vi "HFRR ADV v11.vi"() -> ()   [LabVIEW 2025] (continued)
              n2114 = String Subset(string=w2524, offset (0)=15, length (rest)=9 ("length (rest)")) -> (substring=w2553:string)
              n2115 = String Subset(string=w2524, offset (0)=0, length (rest)=14 ("length (rest)")) -> (substring=w2550:string)
              n2116 = String Subset(string=w2524, offset (0)=45, length (rest)=9 ("length (rest)")) -> (substring=w2537:string)
              n2117 = String Subset(string=w2524, offset (0)=65, length (rest)=9 ("length (rest)")) -> (substring=w2543:string)
              n2118 = Fract/Exp String To Number(string=w2526) -> (number=w2523:dbl)  [unwired: 3 in, 1 out]
              n2119 = Fract/Exp String To Number(string=w2547) -> (number=w2545:dbl)  [unwired: 3 in, 1 out]
              n2120 = Fract/Exp String To Number(string=w2532) -> (number=w2530:dbl)  [unwired: 3 in, 1 out]
              n2121 = Fract/Exp String To Number(string=w2528) -> (number=w2527:dbl)  [unwired: 3 in, 1 out]
              n2122 = Fract/Exp String To Number(string=w2553) -> (number=w2544:dbl)  [unwired: 3 in, 1 out]
              n2123 = Fract/Exp String To Number(string=w2550) -> (number=w2546:dbl)  [unwired: 3 in, 1 out]
              n2124 = Fract/Exp String To Number(string=w2537) -> (number=w2534:dbl)  [unwired: 3 in, 1 out]
              n2125 = Fract/Exp String To Number(string=w2543) -> (number=w2540:dbl)  [unwired: 3 in, 1 out]
              n2126 = Add(x=w2540, y=0.0) -> (x+y=w2538:dbl)
            }
            n2127 = String To Path(string=w2383) -> (path=w2481:path)
            n2128 = String To Path(string=w2381) -> (path=w2475:path)
            n2129 = local read "Numeric 11"() -> (w2465:i32)
            n2130 = local read "Numeric 13"() -> (w2467:i32)
            n2131 = Open/Create/Replace File "Open File"(file path (use dialog)=w2481) -> (refnum out=w2479:refnum<file>, error out=w2478:errorcluster)  [unwired: 5 in, 1 out]
            n2132 = Open/Create/Replace File "Open File"(file path (use dialog)=w2475) -> (refnum out=w2474:refnum<file>, error out=w2473:errorcluster)  [unwired: 5 in, 1 out]
            n2133 = for {
              N: w2465 -> [_]
              tunnel: w2479 -> [w2594]
              tunnel: w2478 -> [w2593]
              tunnel: [w2583] -> w2445 mode=indexing
              tunnel: [w2581] -> w2443 mode=indexing
              tunnel: [w2582] -> w2438 mode=indexing
              tunnel: w2464 -> [_]
              tunnel: [w2575] -> w2440 mode=indexing
              tunnel: [w2571] -> w2416 mode=indexing
              tunnel: [w2567] -> w2391 mode=indexing
              tunnel: [w2563] -> w2372 mode=indexing
              tunnel: [w2558] -> w2330 mode=indexing
              (unwired) TRUE ("line mode (F)")
              n2134 = Read from Text File "Read File"(file (use dialog)=w2594, error in=w2593) -> (text=w2559:string)  [unwired: 2 in, 3 out]
              n2135 = local write "String 7"(w2559) -> ()
              n2136 = String Subset(string=w2559, offset (0)=85, length (rest)=9 ("length (rest)")) -> (substring=w2562:string)
              n2137 = String Subset(string=w2559, offset (0)=35, length (rest)=9 ("length (rest)")) -> (substring=w2584:string)
              n2138 = String Subset(string=w2559, offset (0)=55, length (rest)=9 ("length (rest)")) -> (substring=w2570:string)
              n2139 = String Subset(string=w2559, offset (0)=25, length (rest)=9 ("length (rest)")) -> (substring=w2564:string)
              n2140 = String Subset(string=w2559, offset (0)=45, length (rest)=9 ("length (rest)")) -> (substring=w2572:string)
              n2141 = String Subset(string=w2559, offset (0)=0, length (rest)=14 ("length (rest)")) -> (substring=w2587:string)
              n2142 = String Subset(string=w2559, offset (0)=15, length (rest)=9 ("length (rest)")) -> (substring=w2590:string)
              n2143 = String Subset(string=w2559, offset (0)=65, length (rest)=9 ("length (rest)")) -> (substring=w2576:string)
              n2144 = Fract/Exp String To Number(string=w2562) -> (number=w2558:dbl)  [unwired: 3 in, 1 out]
              n2145 = Fract/Exp String To Number(string=w2584) -> (number=w2582:dbl)  [unwired: 3 in, 1 out]
              n2146 = Fract/Exp String To Number(string=w2570) -> (number=w2567:dbl)  [unwired: 3 in, 1 out]
              n2147 = Fract/Exp String To Number(string=w2564) -> (number=w2563:dbl)  [unwired: 3 in, 1 out]
              n2148 = Fract/Exp String To Number(string=w2572) -> (number=w2571:dbl)  [unwired: 3 in, 1 out]
              n2149 = Fract/Exp String To Number(string=w2587) -> (number=w2583:dbl)  [unwired: 3 in, 1 out]
              n2150 = Fract/Exp String To Number(string=w2590) -> (number=w2581:dbl)  [unwired: 3 in, 1 out]
              n2151 = Fract/Exp String To Number(string=w2576) -> (number=w2579:dbl)  [unwired: 3 in, 1 out]
              n2152 = Add(x=w2579, y=0.0) -> (x+y=w2575:dbl)
            }
            n2153 = for {
              N: w2467 -> [_]
              tunnel: w2474 -> [w2522]
              tunnel: w2473 -> [w2521]
              tunnel: [w2511] -> w2427 mode=indexing
              tunnel: [w2510] -> w2420 mode=indexing
              tunnel: w2464 -> [_]
              tunnel: [w2499] -> w2425 mode=indexing
              tunnel: [w2504] -> w2422 mode=indexing
              tunnel: [w2500] -> w2412 mode=indexing
              tunnel: [w2495] -> w2387 mode=indexing
              tunnel: [w2491] -> w2368 mode=indexing
              tunnel: [w2486] -> w2328 mode=indexing
              (unwired) 1.0 ("x")
              (unwired) TRUE ("line mode (F)")
              n2154 = Read from Text File "Read File"(file (use dialog)=w2522, error in=w2521) -> (text=w2487:string)  [unwired: 2 in, 3 out]
              n2155 = local write "String 12"(w2487) -> ()
              n2156 = String Subset(string=w2487, offset (0)=85, length (rest)=9 ("length (rest)")) -> (substring=w2489:string)
              n2157 = String Subset(string=w2487, offset (0)=35, length (rest)=9 ("length (rest)")) -> (substring=w2512:string)
              n2158 = String Subset(string=w2487, offset (0)=55, length (rest)=9 ("length (rest)")) -> (substring=w2497:string)
              n2159 = String Subset(string=w2487, offset (0)=25, length (rest)=9 ("length (rest)")) -> (substring=w2493:string)
              n2160 = String Subset(string=w2487, offset (0)=45, length (rest)=9 ("length (rest)")) -> (substring=w2502:string)
              n2161 = String Subset(string=w2487, offset (0)=15, length (rest)=9 ("length (rest)")) -> (substring=w2518:string)
              n2162 = String Subset(string=w2487, offset (0)=0, length (rest)=14 ("length (rest)")) -> (substring=w2515:string)
              n2163 = String Subset(string=w2487, offset (0)=65, length (rest)=9 ("length (rest)")) -> (substring=w2505:string)
              n2164 = Fract/Exp String To Number(string=w2489) -> (number=w2486:dbl)  [unwired: 3 in, 1 out]
              n2165 = Fract/Exp String To Number(string=w2512) -> (number=w2510:dbl)  [unwired: 3 in, 1 out]
              n2166 = Fract/Exp String To Number(string=w2497) -> (number=w2495:dbl)  [unwired: 3 in, 1 out]
              n2167 = Fract/Exp String To Number(string=w2493) -> (number=w2491:dbl)  [unwired: 3 in, 1 out]
              n2168 = Fract/Exp String To Number(string=w2502) -> (number=w2500:dbl)  [unwired: 3 in, 1 out]
              n2169 = Fract/Exp String To Number(string=w2518) -> (number=w2499:dbl)  [unwired: 3 in, 1 out]
              n2170 = Fract/Exp String To Number(string=w2515) -> (number=w2511:dbl)  [unwired: 3 in, 1 out]
              n2171 = Fract/Exp String To Number(string=w2505) -> (number=w2508:dbl)  [unwired: 3 in, 1 out]
              n2172 = Add(x=w2508, y=0.0) -> (x+y=w2504:dbl)
            }
            n2173 = Delete From Array(array=w2370, index=0) -> (array with subset deleted=w2343:dbl[])  [unwired: 1 in, 1 out]
            n2174 = Delete From Array(array=w2433, index=0) -> (array with subset deleted=w2406:dbl[])  [unwired: 1 in, 1 out]
            n2175 = Delete From Array(array=w2413, index=0) -> (array with subset deleted=w2401:dbl[])  [unwired: 1 in, 1 out]
            n2176 = Delete From Array(array=w2431, index=0) -> (array with subset deleted=w2432:dbl[])  [unwired: 1 in, 1 out]
            n2177 = call-poly <vilib>:"Mean.vi"("X"=w2343) -> ("mean"=→"КОФ2 4":dbl)  [unwired: 1 out]
            n2178 = call-poly <vilib>:"Mean.vi"("X"=w2406) -> ("mean"=→"КОФ3":dbl)  [unwired: 1 out]
            n2179 = call-poly <vilib>:"Mean.vi"("X"=w2401) -> ("mean"=→"CP3":dbl)  [unwired: 1 out]
            n2180 = Delete From Array(array=w2395, index=0) -> (array with subset deleted=w2322:dbl[])  [unwired: 1 in, 1 out]
            n2181 = Delete From Array(array=w2334, index=0) -> (array with subset deleted=w2321:dbl[])  [unwired: 1 in, 1 out]
            n2182 = Delete From Array(array=w2374, index=0) -> (array with subset deleted=w2345:dbl[])  [unwired: 1 in, 1 out]
            n2183 = Delete From Array(array=w2452, index=0) -> (array with subset deleted=w2407:dbl[])  [unwired: 1 in, 1 out]
            n2184 = Delete From Array(array=w2418, index=0) -> (array with subset deleted=w2403:dbl[])  [unwired: 1 in, 1 out]
            "array w/ subset deleted" <- w2403
            n2185 = Delete From Array(array=w2449, index=0) -> (array with subset deleted=w2450:dbl[])  [unwired: 1 in, 1 out]
            n2186 = call-poly <vilib>:"Mean.vi"("X"=w2345) -> ("mean"=→"КОФ2 2":dbl)  [unwired: 1 out]
            n2187 = call-poly <vilib>:"Mean.vi"("X"=w2407) -> ("mean"=→"КОФ1":dbl)  [unwired: 1 out]
            n2188 = Bundle "Bundle"(w2322, w2321) -> (w2327:cluster{dbl[], dbl[]})  [unwired: 1 in]
            n2189 = Bundle "Bundle"(w2322, w2450) -> (w2314:cluster{dbl[], dbl[]})  [unwired: 1 in]
            n2190 = Delete From Array(array=w2329, index=0) -> (array with subset deleted=w2317:dbl[])  [unwired: 1 in, 1 out]
            n2191 = Delete From Array(array=w2330, index=0) -> (array with subset deleted=w2319:dbl[])  [unwired: 1 in, 1 out]
            n2192 = Delete From Array(array=w2440, index=0) -> (array with subset deleted=w2441:dbl[])  [unwired: 1 in, 1 out]
            n2193 = Delete From Array(array=w2328, index=0) -> (array with subset deleted=w2315:dbl[])  [unwired: 1 in, 1 out]
            n2194 = Delete From Array(array=w2422, index=0) -> (array with subset deleted=w2423:dbl[])  [unwired: 1 in, 1 out]
            n2195 = Delete From Array(array=w2447, index=0) -> (array with subset deleted=w2353:dbl[])  [unwired: 1 in, 1 out]
            n2196 = Delete From Array(array=w2393, index=0) -> (array with subset deleted=w2349:dbl[])  [unwired: 1 in, 1 out]
            n2197 = Delete From Array(array=w2429, index=0) -> (array with subset deleted=w2351:dbl[])  [unwired: 1 in, 1 out]
            n2198 = Delete From Array(array=w2389, index=0) -> (array with subset deleted=w2347:dbl[])  [unwired: 1 in, 1 out]
            n2199 = Delete From Array(array=w2438, index=0) -> (array with subset deleted=w2352:dbl[])  [unwired: 1 in, 1 out]
            n2200 = Delete From Array(array=w2391, index=0) -> (array with subset deleted=w2348:dbl[])  [unwired: 1 in, 1 out]
            n2201 = Delete From Array(array=w2372, index=0) -> (array with subset deleted=w2344:dbl[])  [unwired: 1 in, 1 out]
            n2202 = Delete From Array(array=w2416, index=0) -> (array with subset deleted=w2402:dbl[])  [unwired: 1 in, 1 out]
            n2203 = Delete From Array(array=w2443, index=0) -> (array with subset deleted=w2404:dbl[])  [unwired: 1 in, 1 out]
            n2204 = Delete From Array(array=w2420, index=0) -> (array with subset deleted=w2350:dbl[])  [unwired: 1 in, 1 out]
            n2205 = Delete From Array(array=w2387, index=0) -> (array with subset deleted=w2346:dbl[])  [unwired: 1 in, 1 out]
            n2206 = Delete From Array(array=w2368, index=0) -> (array with subset deleted=w2342:dbl[])  [unwired: 1 in, 1 out]
            n2207 = Delete From Array(array=w2412, index=0) -> (array with subset deleted=w2400:dbl[])  [unwired: 1 in, 1 out]
            n2208 = Delete From Array(array=w2425, index=0) -> (array with subset deleted=w2405:dbl[])  [unwired: 1 in, 1 out]
            n2209 = Delete From Array(array=w2435, index=0) -> (array with subset deleted=w2318:dbl[])  [unwired: 1 in, 1 out]
            n2210 = Delete From Array(array=w2445, index=0) -> (array with subset deleted=w2320:dbl[])  [unwired: 1 in, 1 out]
            n2211 = Delete From Array(array=w2427, index=0) -> (array with subset deleted=w2316:dbl[])  [unwired: 1 in, 1 out]
            n2212 = Bundle "Bundle"(w2322, w2353) -> (w2340:cluster{dbl[], dbl[]})  [unwired: 1 in]
            n2213 = Bundle "Bundle"(w2322, w2407) -> (w2341:cluster{dbl[], dbl[]})  [unwired: 1 in]
            n2214 = Bundle "Bundle"(w2353, w2349) -> (w2355:cluster{dbl[], dbl[]})  [unwired: 1 in]
            n2215 = Bundle "Bundle"(w2318, w2317) -> (w2325:cluster{dbl[], dbl[]})  [unwired: 1 in]
            n2216 = Bundle "Bundle"(w2351, w2347) -> (w2357:cluster{dbl[], dbl[]})  [unwired: 1 in]
            n2217 = Bundle "Bundle"(w2318, w2351) -> (w2461:cluster{dbl[], dbl[]})  [unwired: 1 in]
            n2218 = Bundle "Bundle"(w2318, w2347) -> (w2385:cluster{dbl[], dbl[]})  [unwired: 1 in]
            n2219 = Bundle "Bundle"(w2318, w2406) -> (w2471:cluster{dbl[], dbl[]})  [unwired: 1 in]
            n2220 = Bundle "Bundle"(w2318, w2401) -> (w2409:cluster{dbl[], dbl[]})  [unwired: 1 in]
            n2221 = Bundle "Bundle"(w2318, w2432) -> (w2456:cluster{dbl[], dbl[]})  [unwired: 1 in]
            n2222 = Bundle "Bundle"(w2352, w2348) -> (w2356:cluster{dbl[], dbl[]})  [unwired: 1 in]
            n2223 = Bundle "Bundle"(w2320, w2319) -> (w2326:cluster{dbl[], dbl[]})  [unwired: 1 in]
            n2224 = Bundle "Bundle"(w2320, w2352) -> (w2463:cluster{dbl[], dbl[]})  [unwired: 1 in]
            n2225 = Bundle "Bundle"(w2320, w2348) -> (w2386:cluster{dbl[], dbl[]})  [unwired: 1 in]
            n2226 = Bundle "Bundle"(w2320, w2402) -> (w2410:cluster{dbl[], dbl[]})  [unwired: 1 in]
            n2227 = Bundle "Bundle"(w2320, w2404) -> (w2472:cluster{dbl[], dbl[]})  [unwired: 1 in]
            n2228 = Bundle "Bundle"(w2320, w2441) -> (w2454:cluster{dbl[], dbl[]})  [unwired: 1 in]
            n2229 = Bundle "Bundle"(w2350, w2346) -> (w2358:cluster{dbl[], dbl[]})  [unwired: 1 in]
            n2230 = Bundle "Bundle"(w2316, w2315) -> (w2324:cluster{dbl[], dbl[]})  [unwired: 1 in]
            n2231 = Bundle "Bundle"(w2316, w2350) -> (w2462:cluster{dbl[], dbl[]})  [unwired: 1 in]
            n2232 = Bundle "Bundle"(w2316, w2346) -> (w2384:cluster{dbl[], dbl[]})  [unwired: 1 in]
            n2233 = Bundle "Bundle"(w2316, w2400) -> (w2408:cluster{dbl[], dbl[]})  [unwired: 1 in]
            n2234 = Bundle "Bundle"(w2316, w2405) -> (w2470:cluster{dbl[], dbl[]})  [unwired: 1 in]
            n2235 = Bundle "Bundle"(w2316, w2423) -> (w2455:cluster{dbl[], dbl[]})  [unwired: 1 in]
            n2236 = call-poly <vilib>:"Mean.vi"("X"=w2403) -> ("mean"=→"CP1":dbl)  [unwired: 1 out]
            n2237 = call-poly <vilib>:"Mean.vi"("X"=w2344) -> ("mean"=→"КОФ2 3":dbl)  [unwired: 1 out]
            n2238 = call-poly <vilib>:"Mean.vi"("X"=w2402) -> ("mean"=→"CP2":dbl)  [unwired: 1 out]
            n2239 = call-poly <vilib>:"Mean.vi"("X"=w2404) -> ("mean"=→"КОФ2":dbl)  [unwired: 1 out]
            n2240 = call-poly <vilib>:"Mean.vi"("X"=w2342) -> ("mean"=→"КОФ2 5":dbl)  [unwired: 1 out]
            n2241 = call-poly <vilib>:"Mean.vi"("X"=w2400) -> ("mean"=→"CP4":dbl)  [unwired: 1 out]
            n2242 = call-poly <vilib>:"Mean.vi"("X"=w2405) -> ("mean"=→"КОФ4":dbl)  [unwired: 1 out]
            n2243 = Bundle "Bundle"(w2322, w2349) -> (w2313:cluster{dbl[], dbl[]})  [unwired: 1 in]
            n2244 = Bundle "Bundle"(w2322, w2403) -> (w2336:cluster{dbl[], dbl[]})  [unwired: 1 in]
            n2245 = Build Array "Build Array"(w2313, w2336) -> (w2339:cluster{dbl[], dbl[]}[])
            "XY Graph 17" <- w2339
            n2246 = Build Array "Build Array"(w2327, w2326, w2325, w2324) -> (→"Frequency ( Hz )":cluster{dbl[], dbl[]}[])
            n2247 = Build Array "Build Array"(w2355, w2356, w2357, w2358) -> (→"Air Temp ( °C ) vs Humidity ( % RH )":cluster{dbl[], dbl[]}[])
            n2248 = Build Array "Build Array"(w2340, w2463, w2461, w2462) -> (→"Air Temperature  ( °C )":cluster{dbl[], dbl[]}[])
            n2249 = Build Array "Build Array"(w2313, w2386, w2385, w2384) -> (→"Humidity ( %RH )":cluster{dbl[], dbl[]}[])
            n2250 = Build Array "Build Array"(w2341, w2472, w2471, w2470) -> (→"Coefficient Of Friction":cluster{dbl[], dbl[]}[])
            n2251 = Build Array "Build Array"(w2336, w2410, w2409, w2408) -> (→"Sample Temperature ( °C )":cluster{dbl[], dbl[]}[])
            n2252 = Build Array "Build Array"(w2314, w2454, w2456, w2455) -> (→"XY Graph 13":cluster{dbl[], dbl[]}[])
            n2253 = Bundle "Bundle"(w2322, w2345) -> (w2367:cluster{dbl[], dbl[]})  [unwired: 1 in]
            n2254 = Bundle "Bundle"(w2318, w2343) -> (w2365:cluster{dbl[], dbl[]})  [unwired: 1 in]
            n2255 = Bundle "Bundle"(w2320, w2344) -> (w2366:cluster{dbl[], dbl[]})  [unwired: 1 in]
            n2256 = Bundle "Bundle"(w2316, w2342) -> (w2364:cluster{dbl[], dbl[]})  [unwired: 1 in]
            n2257 = Build Array "Build Array"(w2367, w2366, w2365, w2364) -> (→"Stroke ( mm )":cluster{dbl[], dbl[]}[])
            n2258 = local write "XY Graph 16"(w2339) -> ()
          }
          frame #2 {
          }
          frame #3 {
            n2259 = local write "Numeric 8"(0 ("Numeric 8")) -> ()
            n2260 = local write "Numeric 11"(0 ("Numeric 11")) -> ()
            n2261 = local write "Numeric 12"(0 ("Numeric 12")) -> ()
            n2262 = local write "Numeric 13"(0 ("Numeric 13")) -> ()
            n2263 = property on="OPEN" class="Bool (strict)"("Visible"=TRUE) -> ()  [unwired: 2 in, 2 out]
            n2264 = local read "String Control 2"() -> (w2639:string)
            n2265 = local read "String Control 4"() -> (w2638:string)
            n2266 = local read "String Control 6"() -> (w2637:string)
            n2267 = local read "String Control 8"() -> (w2636:string)
            n2268 = Match Pattern(string=w2639, regular expression="Samples / cycle :- ") -> (after substring=w2653:string)  [unwired: 1 in, 3 out]
            n2269 = Match Pattern(string=w2639, regular expression="Frequency :- ") -> (after substring=w2672:string)  [unwired: 1 in, 3 out]
            n2270 = Match Pattern(string=w2638, regular expression="Samples / cycle :- ") -> (after substring=w2649:string)  [unwired: 1 in, 3 out]
            n2271 = Match Pattern(string=w2638, regular expression="Frequency :- ") -> (after substring=w2667:string)  [unwired: 1 in, 3 out]
            n2272 = Match Pattern(string=w2637, regular expression="Samples / cycle :- ") -> (after substring=w2645:string)  [unwired: 1 in, 3 out]
            n2273 = Match Pattern(string=w2637, regular expression="Frequency :- ") -> (after substring=w2662:string)  [unwired: 1 in, 3 out]
            n2274 = Match Pattern(string=w2636, regular expression="Samples / cycle :- ") -> (after substring=w2641:string)  [unwired: 1 in, 3 out]
            n2275 = Match Pattern(string=w2636, regular expression="Frequency :- ") -> (after substring=w2657:string)  [unwired: 1 in, 3 out]
            n2276 = String Subset(string=w2653, length (rest)=6 ("length (rest)")) -> (substring=w2655:string)  [unwired: 1 in]
            n2277 = String Subset(string=w2672, length (rest)=9 ("length (rest)")) -> (substring=w2674:string)  [unwired: 1 in]
            n2278 = String Subset(string=w2649, length (rest)=6 ("length (rest)")) -> (substring=w2651:string)  [unwired: 1 in]
            n2279 = String Subset(string=w2667, length (rest)=9 ("length (rest)")) -> (substring=w2669:string)  [unwired: 1 in]
            n2280 = String Subset(string=w2645, length (rest)=6 ("length (rest)")) -> (substring=w2647:string)  [unwired: 1 in]
            n2281 = String Subset(string=w2662, length (rest)=9 ("length (rest)")) -> (substring=w2664:string)  [unwired: 1 in]
            n2282 = String Subset(string=w2641, length (rest)=6 ("length (rest)")) -> (substring=w2643:string)  [unwired: 1 in]
            n2283 = String Subset(string=w2657, length (rest)=9 ("length (rest)")) -> (substring=w2659:string)  [unwired: 1 in]
            n2284 = Fract/Exp String To Number(string=w2655) -> (number=w2635:dbl)  [unwired: 3 in, 1 out]
            n2285 = Fract/Exp String To Number(string=w2674) -> (number=w2675:dbl)  [unwired: 3 in, 1 out]
            n2286 = Fract/Exp String To Number(string=w2651) -> (number=w2634:dbl)  [unwired: 3 in, 1 out]
            n2287 = Fract/Exp String To Number(string=w2669) -> (number=w2670:dbl)  [unwired: 3 in, 1 out]
            n2288 = Fract/Exp String To Number(string=w2647) -> (number=w2633:dbl)  [unwired: 3 in, 1 out]
            n2289 = Fract/Exp String To Number(string=w2664) -> (number=w2665:dbl)  [unwired: 3 in, 1 out]
            n2290 = Fract/Exp String To Number(string=w2643) -> (number=w2632:dbl)  [unwired: 3 in, 1 out]
            n2291 = Fract/Exp String To Number(string=w2659) -> (number=w2660:dbl)  [unwired: 3 in, 1 out]
            n2292 = local write "sample1"(w2635) -> ()
            n2293 = local write "freq1"(w2675) -> ()
            n2294 = local write "sample2"(w2634) -> ()
            n2295 = local write "freq2"(w2670) -> ()
            n2296 = local write "sample3"(w2633) -> ()
            n2297 = local write "freq3"(w2665) -> ()
            n2298 = local write "sample4"(w2632) -> ()
            n2299 = local write "freq 4"(w2660) -> ()
          }
        }
      }
    }
    n2300 = case shown="True" w2122 {
      selector: w2122 -> [_ w2251]
      frame False {
      }
      frame True {
        n2301 = Not(x=w2251) -> (.not. x?=w2247:bool)
        n2302 = local write "service 3"(w2247) -> ()
        n2303 = local write "OPEN 6"(w2247) -> ()
        n2304 = call <vilib>:"System Exec.vi"("wait until completion? (T)"=TRUE, "command line"="C:\\LAB-IQ\\Scar View.exe") -> ("error out"=→"error out 5":errorcluster)  [unwired: 6 in, 3 out]
      }
    }
    n2305 = case shown="\"Acquire\", Default" w2134 {
      frame "Acquire", Default {
        w3174 = 0.2 ("y")
        w3179 = 1.0 ("y")
        w3180 = 0.8 ("y")
        # "Elapsed time\ncof\nstroke\nAir temp\nTemp\nHumidity"
        n2306 = disable-structure shown="Disabled" {
          frame Disabled {
            n2307 = local read "Flag"() -> (w3197:dbl)
            n2308 = local read "RUN"() -> (w3194:bool)
            n2309 = Not(x=w3194) -> (.not. x?=w3193:bool)
            n2310 = Equal?(x=w3197, y=10.0) -> (x = y?=w3195:bool)
            n2311 = And(x=w3195, y=w3193) -> (x .and. y?=w3192:bool)
            n2312 = case shown="True" w3192 {
              frame False {
              }
              frame True {
                w3198 = FALSE ("Heater Button")
                n2313 = local write "Humidity"(w3198) -> ()
                n2314 = local write "Heater Button"(w3198) -> ()
              }
            }
          }
          frame Enabled {
          }
        }
        n2315 = disable-structure shown="Disabled" {
          frame Disabled {
            n2316 = case shown="True" {
              selector: _ -> [_ _]
              frame False {
              }
              frame True {
                w3289 = TRUE ("Heater")
                n2317 = local write "Humidity"(w3289) -> ()
                n2318 = local write "Heater Button"(w3289) -> ()
                n2319 = local read "TEST STANDARD"() -> (w3292:T3)
                n2320 = local read "TEST STANDARD"() -> (w3287:T3)
                n2321 = Equal?(x=w3292, y=enum16{"ASTM D6079", "ISO 12156", "Custom"}."ISO 12156" ("Test Standard")) -> (x = y?=w3290:bool)
                n2322 = Equal?(x=w3287, y=enum16{"ASTM D6079", "ISO 12156", "Custom"}."ASTM D6079" ("Test Standard")) -> (x = y?=w3286:bool)
                n2323 = case shown="True" w3290 {
                  frame False {
                  }
                  frame True {
                    n2324 = local write "Heater"(TRUE ("Heater")) -> ()
                    n2325 = local write "airtempflg"(FALSE ("airtempflg")) -> ()
                  }
                }
                n2326 = case shown="True" w3286 {
                  frame False {
                  }
                  frame True {
                    n2327 = local write "Heater"(FALSE ("Heater")) -> ()
                    n2328 = local write "airtempflg"(TRUE ("airtempflg")) -> ()
                  }
                }
              }
            }
          }
          frame Enabled {
          }
        }
        n2329 = stacked-sequence {
          frame #0 {
            n2330 = case shown="True" "RST FF" {
              frame False {
              }
              frame True {
                w3355 = 0.0 ("X Scale.Range:Maximum")
                n2331 = property on="Frictional Force ( N )" class="WFChart (strict)"("XScale.Maximum"=600.0 ("X Scale.Range:Maximum"), "XScale.Minimum"=w3355, "YScale.Maximum"=10.0 ("Y Scale.Range:Maximum"), "YScale.Minimum"=w3355) -> ()  [unwired: 2 in, 2 out]
              }
            }
          }
          frame #1 {
            n2332 = case shown="True" "RST TEMP" {
              frame False {
              }
              frame True {
                n2333 = property on="Temperature ( Deg C )" class="WFChart (strict)"("XScale.Minimum"=0.0 ("X Scale.Range:Minimum"), "XScale.Maximum"=600.0 ("X Scale.Range:Maximum"), "YScale.Minimum"=0.0 ("Y Scale.Range:Minimum"), "YScale.Maximum"=100.0 ("Y Scale.Range:Maximum")) -> ()  [unwired: 2 in, 2 out]
              }
            }
          }
          frame #2 {
            n2334 = case shown="True" "RSTCOF" {
              frame False {
              }
              frame True {
                n2335 = property on="Coefficient of Friction" class="WFChart (strict)"("XScale.Minimum"=0.0 ("X Scale.Range:Minimum"), "XScale.Maximum"=600.0 ("X Scale.Range:Maximum"), "YScale.Maximum"=1.0 ("X Scale.Range:Minimum"), "YScale.Minimum"=0.0 ("X Scale.Range:Minimum")) -> ()  [unwired: 2 in, 2 out]
              }
            }
          }
          frame #3 {
            n2336 = case shown="True" "RSTCOF 2" {
              frame False {
              }
              frame True {
                (unwired) 100.0 ("Y Scale.Range:Maximum")
                (unwired) 0.0 ("Y Scale.Range:Minimum")
                (unwired) 600.0 ("X Scale.Range:Maximum")
                (unwired) 0.0 ("X Scale.Range:Minimum")
              }
            }
          }
          frame #4 {
            n2337 = case shown="True" "RSTCOF 3" {
              frame False {
              }
              frame True {
                n2338 = property on="Electrical Contact Resistance ( % )" class="WFChart (strict)"("XScale.Minimum"=0.0 ("X Scale.Range:Minimum"), "XScale.Maximum"=600.0 ("X Scale.Range:Maximum"), "YScale.Minimum"=0.0 ("Y Scale.Range:Minimum"), "YScale.Maximum"=100.0 ("Y Scale.Range:Maximum")) -> ()  [unwired: 2 in, 2 out]
              }
            }
          }
        }
        n2339 = disable-structure shown="Disabled" {
          frame Disabled {
            n2340 = case shown="True" {
              selector: _ -> [_ _]
              frame False {
              }
              frame True {
                n2341 = local read "zflag 2"() -> (w3256:dbl)
                n2342 = local read "yflag"() -> (w3258:dbl)
                n2343 = Equal?(x=w3258, y=2.0 ("tflag")) -> (x = y?=w3260:bool)
                n2344 = Equal?(x=w3256, y=3.0 ("tflag")) -> (x = y?=w3259:bool)
                n2345 = And(x=w3260, y=w3259) -> (x .and. y?=w3254:bool)
                n2346 = case shown="True" w3254 {
                  frame False {
                  }
                  frame True {
                    w3285 = 0.0 ("zflag")
                    n2347 = local write "zflag"(w3285) -> ()
                    n2348 = local write "zflag 2"(w3285) -> ()
                    n2349 = Delete(path (use dialog)=path "C:/LAB-IQ-NXT/WO 2449 TT.sig" ("file path (dialog if empty)")) -> (deleted path=w3284:path)  [unwired: 4 in, 2 out]
                    n2350 = Delete(path (use dialog)=path "C:/LAB-IQ-NXT/WO 2449 TRH.sig" ("file path (dialog if empty)")) -> (deleted path=w3279:path)  [unwired: 4 in, 2 out]
                    n2351 = local read "SEN.RUN HRS"() -> (w3271:dbl)
                    n2352 = local read "SENSOR TIME"() -> (w3269:dbl)
                    n2353 = call <vilib>:"compatOverwrite.vi"("overwrite (F)"=TRUE) -> ("overwrite?"=w3261:T26)
                    n2354 = call <vilib>:"compatOverwrite.vi"("overwrite (F)"=TRUE) -> ("overwrite?"=w3265:T26)
                    n2355 = local read "Total No. of Tests"() -> (w3272:dbl)
                    n2356 = Add(x=w3269, y=w3271) -> (x+y=w3270:dbl)
                    "SEN.RUN HRS" <- w3270
                    n2357 = Open/Create/Replace File(file path (use dialog)=w3284, operation (0:open)=w3261) -> (refnum out=w3262:refnum<file>, error out=w3263:errorcluster)  [unwired: 4 in, 1 out]
                    n2358 = Open/Create/Replace File(file path (use dialog)=w3279, operation (0:open)=w3265) -> (refnum out=w3266:refnum<file>, error out=w3267:errorcluster)  [unwired: 4 in, 1 out]
                    n2359 = Deny Access(4:w3263, 6:T24."deny none" ("deny mode (2)"), 7:w3262) -> (3:w3283:refnum<file>)  [unwired: 1 out]
                    n2360 = Deny Access(4:w3267, 6:T24."deny none" ("deny mode (2)"), 7:w3266) -> (3:w3275:refnum<file>)  [unwired: 1 out]
                    n2361 = Number To Decimal String(number=w3272) -> (decimal integer string=w3280:string)  [unwired: 1 in]
                    n2362 = Number To Decimal String(number=w3270) -> (decimal integer string=w3276:string)  [unwired: 1 in]
                    n2363 = Write to Binary File(file (use dialog)=w3283, data=w3280, 5:FALSE ("prepend array or string size? (T)")) -> ()  [unwired: 3 in, 3 out]
                    n2364 = Write to Binary File(file (use dialog)=w3275, data=w3276, 5:FALSE ("prepend array or string size? (T)")) -> ()  [unwired: 3 in, 3 out]
                  }
                }
              }
            }
          }
          frame Enabled {
          }
        }
        n2365 = local read "RUN"() -> (w3183:bool)
        n2366 = local read "run replace"() -> (w3187:bool)
        n2367 = local read "run replace"() -> (w3186:bool)
        n2368 = case shown="True" w3183 {
          frame False {
            n2369 = local write "run replace"(FALSE ("run replace")) -> ()
          }
          frame True {
            "run replace" <- TRUE ("run replace")
          }
        }
        n2370 = local read "RUN"() -> (w3191:bool)
        n2371 = local read "Set Temp"() -> (w3153:dbl)
        n2372 = local read "SetTemp"() -> (w3155:dbl)
        n2373 = case shown="False" w3191 {
          tunnel: [FALSE ("TEST RUNNING") TRUE ("TEST RUNNING")] -> w3190
          frame False {
            w3374 = 0.0 ("Flag")
            n2374 = local write "Elapsed time"(0.0 ("elapsedtime")) -> ()
            n2375 = local write "Time Remaining"(w3374) -> ()
            n2376 = local write "Flag"(w3374) -> ()
            n2377 = local write "Remaining Time"(w3374) -> ()
          }
          frame True {
            n2378 = local write "Flag"(10.0 ("Flag")) -> ()
          }
        }
        n2379 = case shown="False" w3187 {
          frame False {
            n2380 = local read "zflag"() -> (→"zflag 2":dbl)
            n2381 = local write "yflag"(2.0 ("tflag")) -> ()
            n2382 = local write "FLAG 4"(0.0 ("FLAG")) -> ()
          }
          frame True {
            n2383 = local write "yflag"(1.0 ("tflag")) -> ()
            n2384 = local write "zflag"(3.0 ("zflag")) -> ()
          }
        }
        n2385 = local read "acq 2"() -> (w3185:bool)
        n2386 = local read "AIR TEMP"() -> (w3148:dbl)
        n2387 = local read "Amb temp"() -> (w3152:dbl)
        n2388 = case shown="True" "Save & Continue" {
          frame False {
          }
          frame True {
            "acq 2" <- TRUE ("acq 2")
          }
        }
        n2389 = local read "Set Rh"() -> (w3154:dbl)
        n2390 = Add(x=w3155, y=w3180) -> (x+y=w3181:dbl)
        n2391 = Subtract(x=w3155, y=w3180) -> (x-y=w3182:dbl)
        n2392 = Add(x=w3153, y=w3174) -> (x+y=w3175:dbl)
        n2393 = Subtract(x=w3153, y=w3174) -> (x-y=w3176:dbl)
        n2394 = And(x=w3185, y=w3186) -> (x .and. y?=w3184:bool)
        n2395 = Greater Or Equal?(x=w3148, y=15.0) -> (x >= y?=w3149:bool)
        "powstat" <- w3149
        n2396 = local read "Humidity ( %RH )"() -> (w3151:dbl)
        n2397 = case shown="True" "Save & Continue" {
          frame False {
          }
          frame True {
            n2398 = while {
              tunnel: "0123456789abcdefghijklmnopqrstuvwxyzABCDEFGHIJKLMNOPQRSTUVWXYZ" ("string 2") -> [w3345]
              shift-right: [w3343] -> w3338
              shift-left: "" -> [w3342]
              i -> [w3352]
              stop <- w3351 stop-if-true
              n2399 = Random Number (0-1)() -> (number: 0 to 1=w3346:dbl)
              n2400 = Multiply(x=w3346, y=62.0) -> (x*y=w3348:dbl)
              n2401 = Decrement(x="Length") -> (x-1=w3341:i16)
              n2402 = To Word Integer(number=w3348) -> (16bit integer=w3349:i16)
              n2403 = String Subset(string=w3345, offset (0)=w3349, length (rest)=1 ("length (rest)")) -> (substring=w3344:string)
              n2404 = Greater Or Equal?(x=w3352, y=w3341) -> (x >= y?=w3351:bool)
              n2405 = Concatenate Strings(w3344, w3342) -> (w3343:string)
            }
            n2406 = local write "UUID"(w3338) -> ()
          }
        }
        n2407 = In Range and Coerce(upper limit=w3181, x=w3152, lower limit=w3182) -> (In Range?=w3171:bool)  [unwired: 1 out]
        n2408 = Add(x=w3154, y=w3179) -> (x+y=w3178:dbl)
        n2409 = Subtract(x=w3154, y=w3179) -> (x-y=w3177:dbl)
        n2410 = local read "TEMP"() -> (w3150:dbl)
        n2411 = case shown="True" "Save & Continue" {
          frame False {
          }
          frame True {
            n2412 = local read "Operator ID"() -> (w3694:string)
            n2413 = local read "FILE"() -> (w3700:string)
            n2414 = String Length(string=w3700) -> (length=w3698:i32)
            n2415 = String Length(string=w3694) -> (length=w3695:i32)
            n2416 = Greater?(x=w3698, y=0) -> (0:w3697:bool)
            n2417 = Greater?(x=w3695, y=0) -> (0:w3693:bool)
            n2418 = And(x=w3697, y=w3693) -> (x .and. y?=w3692:bool)
            n2419 = case shown="True" w3692 {
              frame False {
                n2420 = stacked-sequence {
                  frame #0 {
                    n2421 = One Button Dialog(message="Please Enter a File Name and Operator ID to save data !", button name ("OK")="Ok") -> ()  [unwired: 1 out]
                  }
                  frame #1 {
                    n2422 = local write "Save & Continue"(FALSE ("OK Button")) -> ()
                  }
                }
                n2423 = local write "Save & Continue"(FALSE ("OK Button")) -> ()
              }
              frame True {
                n2424 = stacked-sequence {
                  frame #0 {
                    n2425 = local read "FILE"() -> (w3706:string)
                    n2426 = call "file check.vi"("file name in"=w3706) -> ("file name out"=w3705:string)  [unwired: 9 in, 1 out]
                    n2427 = call <vilib>:"Application Directory.vi"() -> ("Application Directory"=w3716:path)
                    n2428 = Build Path(base path=w3716, name or relative path="data") -> (appended path=w3715:path)
                    n2429 = call <vilib>:"Trim Whitespace.vi"("string"=w3705) -> ("trimmed string"=w3713:string)  [unwired: 1 in]
                    n2430 = call <vilib>:"Trim Whitespace.vi"("string"=w3705) -> ("trimmed string"=w3714:string)  [unwired: 1 in]
                    n2431 = List Folder(path=w3715) -> (folder names=w3711:string[])  [unwired: 3 in, 3 out]
                    n2432 = Match Pattern(string=w3713, regular expression="_(") -> (before substring=w3710:string)  [unwired: 1 in, 3 out]
                    n2433 = for {
                      tunnel: w3711 -> [w3725] mode=indexing
                      tunnel: w3710 -> [w3723]
                      shift-right: [w3721] -> w3708
                      shift-left: bool[] [] -> [w3722]
                      n2434 = Match Pattern(string=w3725, regular expression="_(") -> (before substring=w3724:string)  [unwired: 1 in, 3 out]
                      n2435 = Equal?(x=w3724, y=w3723) -> (x = y?=w3720:bool)
                      n2436 = case shown="True" w3720 {
                        tunnel: w3720 -> [_ w3728]
                        tunnel: w3722 -> [w3727 w3730]
                        tunnel: [w3727 w3729] -> w3721
                        frame False {
                        }
                        frame True {
                          n2437 = Insert Into Array(array=w3730, new element=w3728) -> (w3729:bool[])  [unwired: 1 in]
                        }
                      }
                    }
                    n2438 = Equal?(x=w3711, y=w3710) -> (x = y?=w3719:bool[])
                    n2439 = Or Array Elements(Boolean array=w3719) -> (logical OR=w3718:bool)
                    n2440 = Array Size(array=w3708) -> (size(s)=w3707:i32)
                    n2441 = case shown="True" w3718 {
                      tunnel: w3714 -> [_ w3738]
                      tunnel: w3707 -> [_ w3731]
                      frame False {
                      }
                      frame True {
                        n2442 = Number To Decimal String(number=w3731) -> (decimal integer string=w3734:string)  [unwired: 1 in]
                        n2443 = Search/Split String(string=w3738, search string/char (-)="_(" ("regular expression")) -> (substring before match=w3736:string)  [unwired: 1 in, 2 out]
                        n2444 = Concatenate Strings(w3736, "_(" ("regular expression"), w3734, ")" ("regular expression")) -> (w3732:string)
                        n2445 = local write "FILE"(w3732) -> ()
                      }
                    }
                  }
                  frame #1 {
                    w3740 = 0.0
                    w3753 = cluster{"y":dbl, dbl, "y":dbl}[] [] ("History Data")
                    w3754 = FALSE ("Heater Button")
                    (unwired) ")!" ("string")
                    (unwired) ")" ("string")
                    w3752 = dbl[] [] ("History Data")
                    w3758 = "\r"
                    # "C:\\WinDucom\\Data\\"
                    # "C:\\LAB-IQ-NXT\\data"
                    n2446 = local write "Humidity ( %RH )"(w3740) -> ()
                    n2447 = local write "Frequency ( Hz )"(w3740) -> ()
                    n2448 = local write "Stroke 3"(w3740) -> ()
                    n2449 = local write "speedop"(0.0 ("PIDclk 2")) -> ()
                    n2450 = local write "Set Temp 2"(65.0 ("Set Temp 2")) -> ()
                    n2451 = local write "AIR TEMP"(w3740) -> ()
                    n2452 = local write "clk"(0.0 ("clk")) -> ()
                    n2453 = local write "Stroke 4"(w3740) -> ()
                    n2454 = local write "Stroke"(w3740) -> ()
                    n2455 = local write "COF 3"(w3740) -> ()
                    n2456 = local write "COF 2"(w3740) -> ()
                    n2457 = local write "TEMP"(w3740) -> ()
                    n2458 = local write "ecr 3"(w3740) -> ()
                    n2459 = local write "FF 3"(w3740) -> ()
                    n2460 = local write "FF 2"(w3740) -> ()
                    n2461 = property on="Humidity ( %RH )" class="WFChart (strict)"("History Data"=w3752) -> ()  [unwired: 2 in, 2 out]
                    n2462 = property on="Coefficient of Friction" class="WFChart (strict)"("History Data"=w3752) -> ()  [unwired: 2 in, 2 out]
                    n2463 = property on="Coefficient of Friction" class="WFChart (strict)"("History Data"=w3752) -> ()  [unwired: 2 in, 2 out]
                    n2464 = property on="Frictional Force ( N )" class="WFChart (strict)"("History Data"=w3752) -> ()  [unwired: 2 in, 2 out]
                    n2465 = property on="Electrical Contact Resistance ( % )" class="WFChart (strict)"("History Data"=w3752) -> ()  [unwired: 2 in, 2 out]
                    n2466 = property on="Electrical Contact Resistance ( % )" class="WFChart (strict)"("History Data"=w3752) -> ()  [unwired: 2 in, 2 out]
                    n2467 = property on="Temperature ( Deg C )" class="WFChart (strict)"("History Data"=w3752) -> ()  [unwired: 2 in, 2 out]
                    n2468 = property on="Frictional Force ( N )" class="WFChart (strict)"("History Data"=w3752) -> ()  [unwired: 2 in, 2 out]
                    n2469 = property on="Coefficient of Friction" class="WFChart (strict)"("History Data"=w3752) -> ()  [unwired: 2 in, 2 out]
                    n2470 = property on="Frictional Force ( N )" class="WFChart (strict)"("History Data"=w3752) -> ()  [unwired: 2 in, 2 out]
                    n2471 = property on="Electrical Contact Resistance ( % )" class="WFChart (strict)"("History Data"=w3752) -> ()  [unwired: 2 in, 2 out]
                    n2472 = property on="Temperature ( Deg C )" class="WFChart (strict)"("History Data"=w3752) -> ()  [unwired: 2 in, 2 out]
                    n2473 = property on="Humidity ( %RH )" class="WFChart (strict)"("History Data"=w3752) -> ()  [unwired: 2 in, 2 out]
                    n2474 = property on="Stroke ( mm )" class="WFChart (strict)"("History Data"=w3753) -> ()  [unwired: 2 in, 2 out]
                    n2475 = property on="Stroke ( mm )" class="WFChart (strict)"("History Data"=w3753) -> ()  [unwired: 2 in, 2 out]
                    n2476 = local write "Humidity"(w3754) -> ()
                    n2477 = local write "Heater Button"(w3754) -> ()
                    n2478 = local read "FILE"() -> (w3748:string)
                    n2479 = disable-structure shown="Enabled" {
                      disable-tunnel: [w3793 _] -> w3739
                      frame Enabled {
                        n2480 = local read "NORMAL LOAD"() -> (w3793:dbl)
                      }
                      frame Disabled {
                      }
                    }
                    n2481 = call "file check.vi"("file name in"=w3748) -> ("error out"=w3751:errorcluster, "file name out"=w3745:string)  [unwired: 9 in]
                    n2482 = call "FILE PATH CREATION.vi"("error in"=w3751, "FILE NAME :"=w3745) -> ("FILE OUT"=w3744:path)  [unwired: 8 in, 1 out]
                    n2483 = Concatenate Strings(w3745, ".dgf" ("Substring")) -> (w3750:string)
                    n2484 = Concatenate Strings(w3745, ".duf" ("Substring")) -> (w3746:string)
                    n2485 = Multiply(x=w3739, y=1.0) -> (x*y=w3772:dbl)
                    n2486 = Build Path(base path=w3744, name or relative path=w3750) -> (appended path=w3743:path)
                    n2487 = Build Path(base path=w3744, name or relative path=w3746) -> (appended path=w3742:path)
                    n2488 = Number To Fractional String(number=w3772, width (-)=i16 5, precision (6)=i16 2) -> (F-format string=w3780:string)  [unwired: 1 in]
                    n2489 = local read "Fuel Discription :"() -> (w3768:string)
                    n2490 = local read "Batch Ref Num :"() -> (w3756:string)
                    n2491 = Get Date/Time String(date format (0)=enum16{"short", "long", "abbreviated"}."short") -> (date string=w3791:string, time string=w3788:string)  [unwired: 2 in]
                    n2492 = local read "Remarks :"() -> (w3767:string)
                    n2493 = Concatenate Strings("Load :- " ("Substring"), w3780, " grams ," ("Substring")) -> (w3779:string)
                    n2494 = local read "String 41"() -> (w3759:string)
                    n2495 = Concatenate Strings(w3768) -> (w3769:string)
                    n2496 = Concatenate Strings(w3756) -> (w3755:string)
                    n2497 = Concatenate Strings("tested by") -> (w3763:string)
                    n2498 = Concatenate Strings("(" ("Substring"), w3791, ")" ("Substring"), w3788) -> (w3761:string)
                    "concatenated string" <- w3761
                    n2499 = Concatenate Strings(w3767, "," ("string")) -> (w3766:string)
                    n2500 = Concatenate Strings("  TIME;      COF;       STROKE;     AIR TEMP;  TEMP;  HUMIDITY;  ECR; PID-OUT; FREQUENCY" ("Substring"), "\r") -> (w3775:string)
                    n2501 = Concatenate Strings(w3759, w3758, "Fuel Discription :-" ("Substring"), w3769, w3758, w3779, w3758, "Batch Ref Num :-" ("Substring"), w3755, w3758, " Remarks :- " ("Substring"), w3766, w3758, " Date :- " ("Substring"), w3761, w3758, "Tested By :-" ("Substring"), w3763) -> (w3773:string)
                    "REMARKS" <- w3773
                    n2502 = call <vilib>:"Write Characters To File.vi"("append to file? (new file:F)"=FALSE, "character string"=w3775, "file path (dialog if empty)"=w3743) -> ()  [unwired: 2 in, 1 out]
                    n2503 = call <vilib>:"Write Characters To File.vi"("append to file? (new file:F)"=FALSE, "character string"=w3773, "file path (dialog if empty)"=w3742) -> ()  [unwired: 2 in, 1 out]
                  }
                  frame #2 {
                    n2504 = local write "Cycles elapsed"(0 ("Cycles elapsed")) -> ()
                    n2505 = local write "cyclecount"(0 ("cyclecount")) -> ()
                    n2506 = local write "Save & Continue"(FALSE ("OK")) -> ()
                    n2507 = local write "autostrtflg"(TRUE ("autostrtflg")) -> ()
                    n2508 = local write "Save"(FALSE ("Save")) -> ()
                    n2509 = Get Date/Time In Seconds() -> (seconds since 1Jan1904=w3798:timestamp)
                    n2510 = To Double Precision Float(number=w3798) -> (double precision float=w3797:dbl)
                    n2511 = local write "acq timer"(w3797) -> ()
                    n2512 = One Button Dialog(message="Please ensure sample is mounted properly and machine is ready in all aspects for testing !", button name ("OK")="Ok") -> ()  [unwired: 1 out]
                  }
                  frame #3 {
                    n2513 = stacked-sequence {
                      frame #0 {
                        n2514 = local write "Main Dashboard Buttons"(T1."Dashboard" ("Main Dashboard Buttons")) -> ()
                        n2515 = local write "Main Tab"(T2."Acquire" ("Main Tab")) -> ()
                      }
                      frame #1 {
                        n2516 = local write "EVENT LOG"("" ("EVENT LOG")) -> ()
                      }
                      frame #2 {
                        n2517 = Wait (ms)(milliseconds to wait=u32 50) -> ()  [unwired: 1 out]
                      }
                      frame #3 {
                        n2518 = disable-structure shown="Disabled" {
                          frame Disabled {
                            n2519 = local read "EVENT LOG"() -> (w3810:string)
                            n2520 = call "Event Log.vi"("Content"="Test Details", "EVENT LOG"=w3810) -> ("EVENT LOG"=w3809:string)  [unwired: 8 in, 1 out]
                            n2521 = local write "EVENT LOG"(w3809) -> ()
                          }
                          frame Enabled {
                          }
                        }
                      }
                      frame #4 {
                        n2522 = Wait (ms)(milliseconds to wait=u32 50) -> ()  [unwired: 1 out]
                      }
                      frame #5 {
                        n2523 = local read "FILE"() -> (w3812:string)
                        n2524 = Concatenate Strings("File Name :" ("Content"), w3812) -> (w3813:string)
                        n2525 = local read "EVENT LOG"() -> (w3816:string)
                        n2526 = call "Event Log.vi"("Content"=w3813, "EVENT LOG"=w3816) -> ("EVENT LOG"=w3815:string)  [unwired: 8 in, 1 out]
                        n2527 = local write "EVENT LOG"(w3815) -> ()
                      }
                      frame #6 {
                        n2528 = Wait (ms)(milliseconds to wait=u32 50) -> ()  [unwired: 1 out]
                      }
                      frame #7 {
                        n2529 = local read "Batch Ref Num :"() -> (w3818:string)
                        n2530 = Concatenate Strings("Batch Ref No :" ("Content"), w3818) -> (w3819:string)
                        n2531 = local read "EVENT LOG"() -> (w3822:string)
                        n2532 = call "Event Log.vi"("Content"=w3819, "EVENT LOG"=w3822) -> ("EVENT LOG"=w3821:string)  [unwired: 8 in, 1 out]
                        n2533 = local write "EVENT LOG"(w3821) -> ()
                      }
                      frame #8 {
                        n2534 = Wait (ms)(milliseconds to wait=u32 50) -> ()  [unwired: 1 out]
                      }
                      frame #9 {
                        n2535 = local read "tested by"() -> (w3824:string)
                        n2536 = Concatenate Strings("Tested By :" ("Content"), w3824) -> (w3825:string)
                        n2537 = local read "EVENT LOG"() -> (w3828:string)
                        n2538 = call "Event Log.vi"("Content"=w3825, "EVENT LOG"=w3828) -> ("EVENT LOG"=w3827:string)  [unwired: 8 in, 1 out]
                        n2539 = local write "EVENT LOG"(w3827) -> ()
                      }
                      frame #10 {
                        n2540 = Wait (ms)(milliseconds to wait=u32 50) -> ()  [unwired: 1 out]
                      }
                      frame #11 {
                        n2541 = local read "TEST STANDARD"() -> (w3831:T3)
                        n2542 = case shown="\"ASTM D6079\", Default" w3831 {
                          tunnel: ["ASTM D6079" "ISO 12156" "CEC F-096-A-06" "Custom"] -> w3830
                          frame "ASTM D6079", Default {
                          }
                          frame "ISO 12156" {
                          }
                          frame "CEC F-096-A-06" {
                          }
                          frame "Custom" {
                          }
                        }
                        n2543 = Concatenate Strings("Test Standard :" ("Content"), w3830) -> (w3832:string)
                        n2544 = local read "EVENT LOG"() -> (w3835:string)
                        n2545 = call "Event Log.vi"("Content"=w3832, "EVENT LOG"=w3835) -> ("EVENT LOG"=w3834:string)  [unwired: 8 in, 1 out]
                        n2546 = local write "EVENT LOG"(w3834) -> ()
                      }
                      frame #12 {
                        n2547 = Wait (ms)(milliseconds to wait=u32 50) -> ()  [unwired: 1 out]
                      }
                      frame #13 {
                        n2548 = local read "Fuel Discription :"() -> (w3841:string)
                        n2549 = Concatenate Strings("Fuel Description :" ("Content"), w3841) -> (w3842:string)
                        n2550 = local read "EVENT LOG"() -> (w3845:string)
                        n2551 = call "Event Log.vi"("Content"=w3842, "EVENT LOG"=w3845) -> ("EVENT LOG"=w3844:string)  [unwired: 8 in, 1 out]
                        n2552 = local write "EVENT LOG"(w3844) -> ()
                      }
                      frame #14 {
                        n2553 = Wait (ms)(milliseconds to wait=u32 50) -> ()  [unwired: 1 out]
                      }
                      frame #15 {
                        n2554 = local read "Remarks :"() -> (w3847:string)
                        n2555 = Concatenate Strings("Remarks :" ("Content"), w3847) -> (w3848:string)
                        n2556 = local read "EVENT LOG"() -> (w3851:string)
                        n2557 = call "Event Log.vi"("Content"=w3848, "EVENT LOG"=w3851) -> ("EVENT LOG"=w3850:string)  [unwired: 8 in, 1 out]
                        n2558 = local write "EVENT LOG"(w3850) -> ()
                      }
                      frame #16 {
                        n2559 = Wait (ms)(milliseconds to wait=u32 50) -> ()  [unwired: 1 out]
                      }
                      frame #17 {
                        n2560 = local read "Operator ID"() -> (w3853:string)
                        n2561 = Concatenate Strings("Operator ID :" ("Content"), w3853) -> (w3855:string)
                        n2562 = local read "EVENT LOG"() -> (w3857:string)
                        n2563 = call "Event Log.vi"("Content"=w3855, "EVENT LOG"=w3857) -> ("EVENT LOG"=w3856:string)  [unwired: 8 in, 1 out]
                        n2564 = local write "EVENT LOG"(w3856) -> ()
                      }
                      frame #18 {
                        n2565 = Wait (ms)(milliseconds to wait=u32 50) -> ()  [unwired: 1 out]
                      }
                      frame #19 {
                        n2566 = disable-structure shown="Disabled" {
                          frame Disabled {
                            n2567 = local read "EVENT LOG"() -> (w3861:string)
                            n2568 = call "Event Log.vi"("Content"="Test Parameter", "EVENT LOG"=w3861) -> ("EVENT LOG"=w3860:string)  [unwired: 8 in, 1 out]
                            n2569 = local write "EVENT LOG"(w3860) -> ()
                          }
                          frame Enabled {
                          }
                        }
                      }
                      frame #20 {
                        n2570 = Wait (ms)(milliseconds to wait=u32 50) -> ()  [unwired: 1 out]
                      }
                      frame #21 {
                        n2571 = local read "Set Hz"() -> (w3865:dbl)
                        n2572 = Number To Fractional String(number=w3865, precision (6)=i16 2) -> (F-format string=w3864:string)  [unwired: 2 in]
                        n2573 = Concatenate Strings("Set Frequency [Hz] :" ("Content"), w3864) -> (w3867:string)
                        n2574 = local read "EVENT LOG"() -> (w3869:string)
                        n2575 = call "Event Log.vi"("Content"=w3867, "EVENT LOG"=w3869) -> ("EVENT LOG"=w3868:string)  [unwired: 8 in, 1 out]
                        n2576 = local write "EVENT LOG"(w3868) -> ()
                      }
                      frame #22 {
                        n2577 = Wait (ms)(milliseconds to wait=u32 50) -> ()  [unwired: 1 out]
                      }
                      frame #23 {
                        n2578 = local read "NORMAL LOAD"() -> (w3872:dbl)
                        n2579 = Number To Fractional String(number=w3872, precision (6)=i16 2) -> (F-format string=w3873:string)  [unwired: 2 in]
                        n2580 = Concatenate Strings("Applied Load [grams] :" ("Content"), w3873) -> (w3875:string)
                        n2581 = local read "EVENT LOG"() -> (w3877:string)
                        n2582 = call "Event Log.vi"("Content"=w3875, "EVENT LOG"=w3877) -> ("EVENT LOG"=w3876:string)  [unwired: 8 in, 1 out]
                        n2583 = local write "EVENT LOG"(w3876) -> ()
                      }
                      frame #24 {
                        n2584 = Wait (ms)(milliseconds to wait=u32 50) -> ()  [unwired: 1 out]
                      }
                      frame #25 {
                        n2585 = local read "Set Strk"() -> (w3880:dbl)
                        n2586 = Number To Fractional String(number=w3880, precision (6)=i16 2) -> (F-format string=w3881:string)  [unwired: 2 in]
                        n2587 = Concatenate Strings("Set Stroke [mm] :" ("Content"), w3881) -> (w3883:string)
                        n2588 = local read "EVENT LOG"() -> (w3885:string)
                        n2589 = call "Event Log.vi"("Content"=w3883, "EVENT LOG"=w3885) -> ("EVENT LOG"=w3884:string)  [unwired: 8 in, 1 out]
                        n2590 = local write "EVENT LOG"(w3884) -> ()
                      }
                      frame #26 {
                        n2591 = Wait (ms)(milliseconds to wait=u32 50) -> ()  [unwired: 1 out]
                      }
                      frame #27 {
                        n2592 = local read "Set Temp"() -> (w3888:dbl)
                        n2593 = Number To Fractional String(number=w3888, precision (6)=i16 2) -> (F-format string=w3889:string)  [unwired: 2 in]
                        n2594 = Concatenate Strings("Set Temperature [deg C] :" ("Content"), w3889) -> (w3891:string)
                        n2595 = local read "EVENT LOG"() -> (w3893:string)
                        n2596 = call "Event Log.vi"("Content"=w3891, "EVENT LOG"=w3893) -> ("EVENT LOG"=w3892:string)  [unwired: 8 in, 1 out]
                        n2597 = local write "EVENT LOG"(w3892) -> ()
                      }
                      frame #28 {
                        n2598 = Wait (ms)(milliseconds to wait=u32 50) -> ()  [unwired: 1 out]
                      }
                      frame #29 {
                        n2599 = local read "Set Rh"() -> (w3896:dbl)
                        n2600 = Number To Fractional String(number=w3896, precision (6)=i16 2) -> (F-format string=w3897:string)  [unwired: 2 in]
                        n2601 = Concatenate Strings("Set Humidity [%RH] :" ("Content"), w3897) -> (w3899:string)
                        n2602 = local read "EVENT LOG"() -> (w3901:string)
                        n2603 = call "Event Log.vi"("Content"=w3899, "EVENT LOG"=w3901) -> ("EVENT LOG"=w3900:string)  [unwired: 8 in, 1 out]
                        n2604 = local write "EVENT LOG"(w3900) -> ()
                      }
                      frame #30 {
                        n2605 = Wait (ms)(milliseconds to wait=u32 50) -> ()  [unwired: 1 out]
                      }
                      frame #31 {
                        n2606 = local read "test time"() -> (w3904:dbl)
                        n2607 = Number To Fractional String(number=w3904, precision (6)=i16 1) -> (F-format string=w3905:string)  [unwired: 2 in]
                        n2608 = Concatenate Strings("Test Duration [mins] :" ("Content"), w3905) -> (w3907:string)
                        n2609 = local read "EVENT LOG"() -> (w3909:string)
                        n2610 = call "Event Log.vi"("Content"=w3907, "EVENT LOG"=w3909) -> ("EVENT LOG"=w3908:string)  [unwired: 8 in, 1 out]
                        n2611 = local write "EVENT LOG"(w3908) -> ()
                      }
                      frame #32 {
                        w3910 = dbl[] [] ("History Data")
                        w3911 = cluster{"y":dbl, dbl, "y":dbl}[] [] ("History Data")
                        w3912 = FALSE ("Visible")
                        n2612 = property on="Stroke ( mm )" class="WFChart (strict)"("History Data"=w3911) -> ()  [unwired: 2 in, 2 out]
                        n2613 = property on="Humidity ( %RH )" class="WFChart (strict)"("History Data"=w3910) -> ()  [unwired: 2 in, 2 out]
                        n2614 = property on="Temperature ( Deg C )" class="WFChart (strict)"("History Data"=w3910) -> ()  [unwired: 2 in, 2 out]
                        n2615 = property on="Electrical Contact Resistance ( % )" class="WFChart (strict)"("History Data"=w3910) -> ()  [unwired: 2 in, 2 out]
                        n2616 = property on="Coefficient of Friction" class="WFChart (strict)"("History Data"=w3910) -> ()  [unwired: 2 in, 2 out]
                        n2617 = property on="Frictional Force ( N )" class="WFChart (strict)"("History Data"=w3910) -> ()  [unwired: 2 in, 2 out]
                        n2618 = property on="Coefficient of Friction" class="WFChart (strict)"("History Data"=w3910) -> ()  [unwired: 2 in, 2 out]
                        n2619 = property on="Frictional Force ( N )" class="WFChart (strict)"("History Data"=w3910) -> ()  [unwired: 2 in, 2 out]
                        n2620 = property on="Electrical Contact Resistance ( % )" class="WFChart (strict)"("History Data"=w3910) -> ()  [unwired: 2 in, 2 out]
                        n2621 = property on="Humidity ( %RH )" class="WFChart (strict)"("History Data"=w3910) -> ()  [unwired: 2 in, 2 out]
                        n2622 = property on="Stroke ( mm )" class="WFChart (strict)"("History Data"=w3911) -> ()  [unwired: 2 in, 2 out]
                        n2623 = property on="Temperature ( Deg C )" class="WFChart (strict)"("History Data"=w3910) -> ()  [unwired: 2 in, 2 out]
                        n2624 = property on="Service Password Log" class="Str"("Visible"=w3912) -> ()  [unwired: 2 in, 2 out]
                        n2625 = property on="Password 3" class="Clust (strict)"("Visible"=w3912) -> ()  [unwired: 2 in, 2 out]
                      }
                    }
                    "TEST FILE NAM,E SAVED" <- TRUE ("TEST FILE NAM,E SAVED")
                  }
                }
              }
            }
          }
        }
        n2626 = case shown="True" w3184 {
          frame False {
            n2627 = local write "tfalg"(0.0 ("tfalg")) -> ()
          }
          frame True {
            n2628 = local read "tfalg"() -> (w3329:dbl)
            n2629 = Equal?(x=w3329, y=0.0) -> (x = y?=w3330:bool)
            n2630 = case shown="True" w3330 {
              frame False {
              }
              frame True {
                n2631 = local read "Total No. of Tests"() -> (w3333:dbl)
                n2632 = local write "tfalg"(1.0 ("tfalg")) -> ()
                n2633 = local write "acq 2"(FALSE ("acq 2")) -> ()
                n2634 = Wait (ms)(milliseconds to wait=u32 200) -> ()  [unwired: 1 out]
                n2635 = Increment(x=w3333) -> (x+1=w3332:dbl)
                n2636 = local write "Total No. of Tests"(w3332) -> ()
              }
            }
          }
        }
        n2637 = local write "Test \nStatus"(w3190) -> ()
        n2638 = local write "st enable"(w3190) -> ()
        n2639 = local write "PWR"(w3190) -> ()
        n2640 = local write "Save"(w3190) -> ()
        n2641 = local read "Main Tab"() -> (w3147:T2)
        n2642 = case shown="True" w3171 {
          tunnel: [FALSE ("RUN") TRUE ("RUN")] -> w3170
          tunnel: [_ 1] -> w3163
          frame False {
          }
